vi "MemberExcuseNote.vi"() -> ()   [LabVIEW 2015, in "Member_Actor.lvlib"]
uses:
  Member_Actor.lvlib
  ExcuseNote/ExcuseNote.lvclass
  <vilib>/Utility/error.llb/Error Cluster From Error Code.vi
  <vilib>/ErrorRing/Error Ring.xnode
panel:
  in  "ExcuseNote":T1
  in  "提交":bool
  in  "Stop":bool
  out "Member_Actor.lvlib:ExcuseNote.lvclass":refnum<class "ExcuseNote.lvclass">
  in  "Member_Actor.lvlib:ExcuseNote.lvclass":refnum<class "ExcuseNote.lvclass">
  # "-"
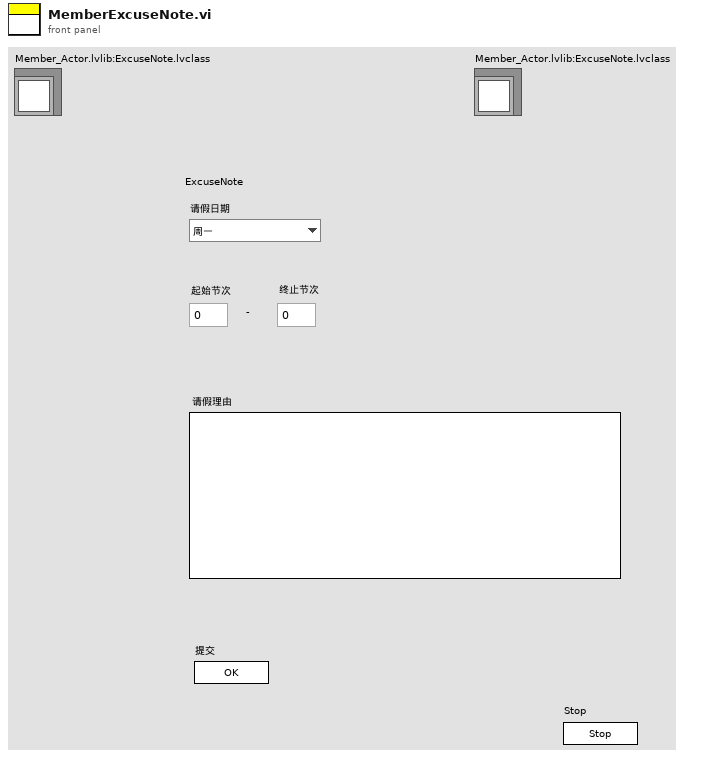
[diagram p1: front panel]
types:
  T1 = cluster{"请假日期":enum16{"周一", "周二", "周三", "周四", "周五", "周六", "周日"}, "起始节次":i32, "终止节次":i32, "请假理由":string}
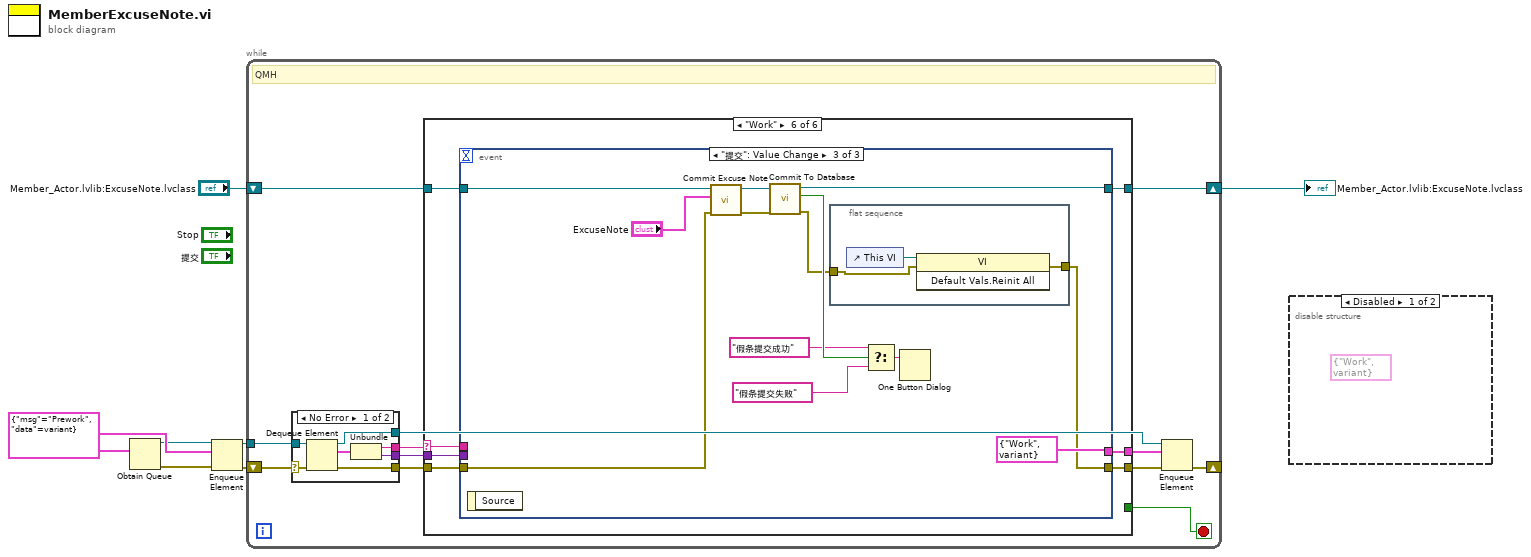
[diagram p0: block diagram]
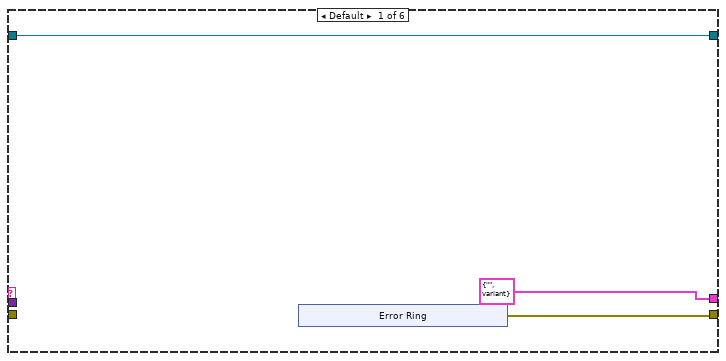
[diagram p3: hidden frame]
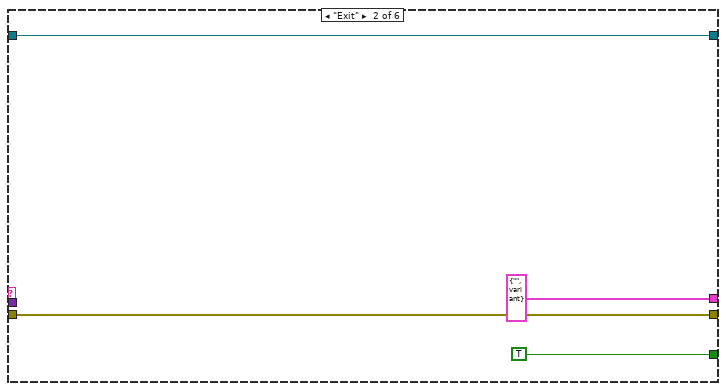
[diagram p4: hidden frame]
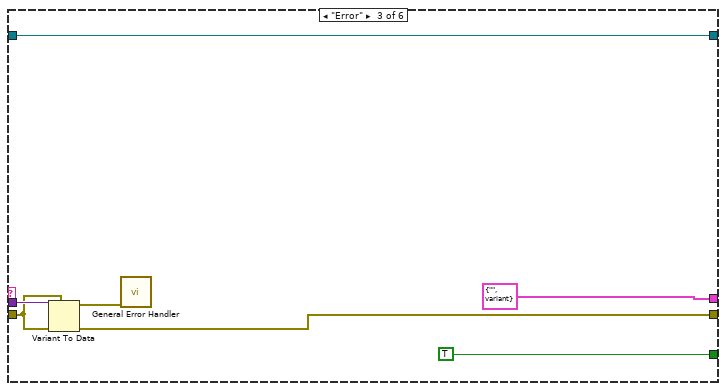
[diagram p5: hidden frame]
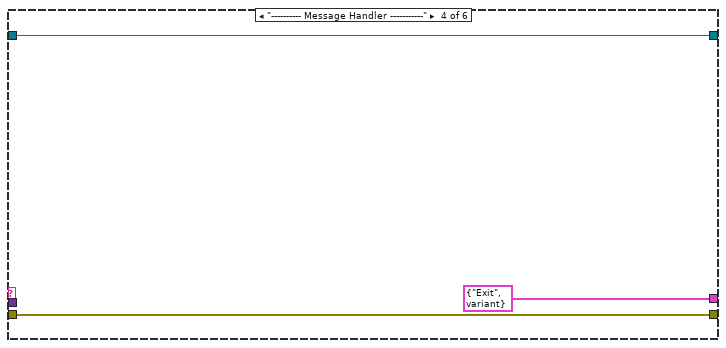
[diagram p6: hidden frame]
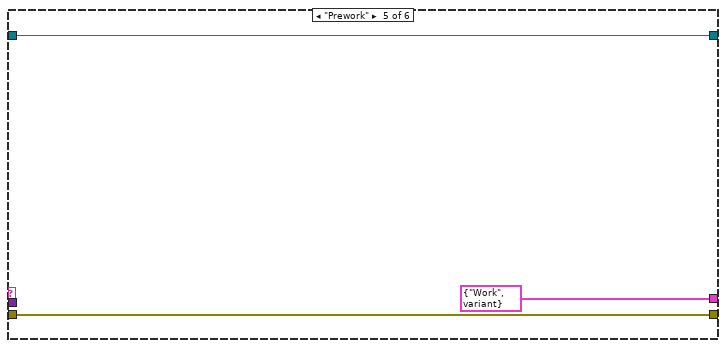
[diagram p7: hidden frame]
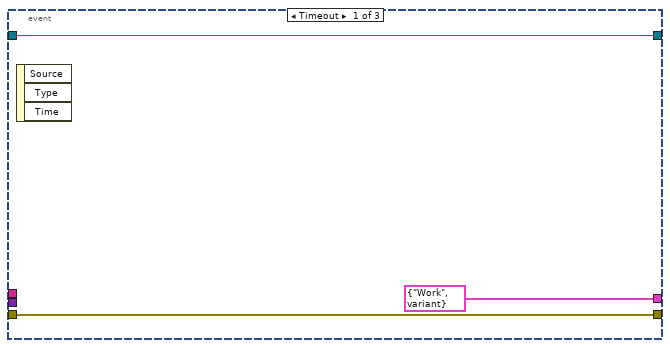
[diagram p8: hidden frame]
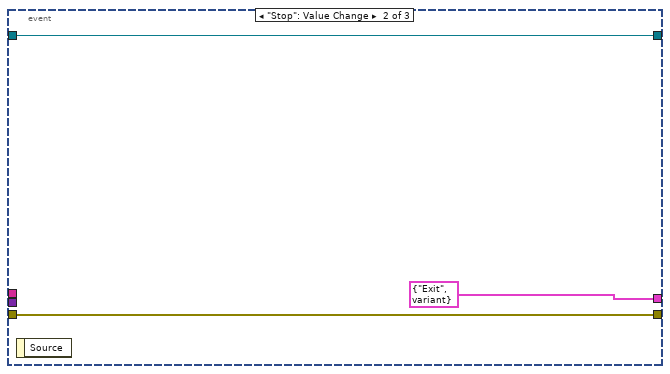
[diagram p9: hidden frame]
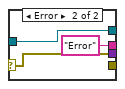
[diagram p10: hidden frame]
diagram:
  w5 = cluster{"msg":string, "data":variant} {"msg"="Prework", "data"=variant}
  n1 = Obtain Queue(element data type=w5) -> (queue out=w3:refnum<queue>, error out=w4:errorcluster)  [unwired: 4 in, 1 out]
  n2 = Enqueue Element(queue=w3, element=w5, error in (no error)=w4) -> (queue out=w6:refnum<queue>, error out=w7:errorcluster)  [unwired: 1 in, 1 out]
  n3 = while {
    tunnel: w6 -> [w18]
    shift-right: [w13] -> _
    shift-left: w7 -> [w19]
    shift-right: [w8] -> w1
    shift-left: "Member_Actor.lvlib:ExcuseNote.lvclass" -> [w9]
    stop <- w10 stop-if-true
    # "QMH"
    n4 = case shown="No Error" w19 {
      selector: w19 -> [w79 w83]
      tunnel: w18 -> [w80 w81]
      tunnel: [w78 _] -> w17
      tunnel: [w76 "Error" ("msg")] -> w16
      tunnel: [w75 w83] -> w15
      tunnel: [w74 w81] -> w12
      frame No Error {
        n5 = Dequeue Element(queue=w80, error in (no error)=w79) -> (queue out=w74:refnum<queue>, element=w77:cluster{"msg":string, "data":variant}, error out=w78:errorcluster)  [unwired: 1 in, 1 out]
        n6 = Unbundle(w77) -> ("msg"=w76:string, "data"=w75:variant)
      }
      frame Error {
      }
    }
    n7 = case shown="\"Work\"" w16 {
      selector: w16 -> [_ _ _ _ _ w49]
      tunnel: w17 -> [_ w31 w37 w41 w43 w51]
      tunnel: w15 -> [_ _ w38 _ _ w50]
      tunnel: [w22 w31 w35 w41 w43 w48] -> w14
      tunnel: [cluster{"msg":string, "data":variant} {"msg"="", "data"=variant} cluster{"msg":string, "data":variant} {"msg"="", "data"=variant} cluster{"msg":string, "data":variant} {"msg"="", "data"=variant} cluster{"msg":string, "data":variant} {"msg"="Exit", "data"=variant} cluster{"msg":string, "data":variant} {"msg"="Work", "data"=variant} w47] -> w11
      tunnel: [_ TRUE TRUE _ _ _] -> w10
      tunnel: w9 -> [w20 w28 w32 w39 w42 w46]
      tunnel: [w20 w28 w32 w39 w42 w45] -> w8
      frame Default {
        n8 = xnode "Error Ring"() -> ("error out"=w22:errorcluster)
      }
      frame "Exit" {
      }
      frame "Error" {
        n9 = Variant To Data(error in=w37, type=w37, Variant=w38) -> (data=w36:errorcluster, error out=w35:errorcluster)
        n10 = call <vilib>:"General Error Handler.vi"("error in (no error)"=w36) -> ()  [unwired: 10 in, 5 out]
      }
      frame "---------- Message Handler -----------" {
      }
      frame "Prework" {
      }
      frame "Work" {
        n11 = event shown="[2] \"提交\": Value Change" {
          selector: _ -> [_ _ _]
          dyn-events: _ -> [_ _ _]
          timeout: _ -> [_ _ _]
          tunnel: w51 -> [w54 w57 w68]
          tunnel: w50 -> [_ _ _]
          tunnel: w49 -> [_ _ _]
          tunnel: [w54 w57 w58] -> w48
          tunnel: [cluster{"msg":string, "data":variant} {"msg"="Work", "data"=variant} cluster{"msg":string, "data":variant} {"msg"="Exit", "data"=variant} cluster{"msg":string, "data":variant} {"msg"="Work", "data"=variant}] -> w47
          tunnel: w46 -> [w52 w55 w70]
          tunnel: [w52 w55 w64] -> w45
          event Timeout {
            n12 = event-data() -> ()  [unwired: 1 in, 3 out]
          }
          event "Stop": Value Change {
            n13 = event-data() -> ()  [unwired: 1 in, 1 out]
          }
          event "提交": Value Change {
            n14 = event-data() -> ()  [unwired: 1 in, 1 out]
            n15 = call "Commit Excuse Note.vi"("error in (no error)"=w68, "ExcuseNote"="ExcuseNote", "ExcuseNote in"=w70) -> ("error out"=w65:errorcluster, "ExcuseNote out"=w66:refnum<class "ExcuseNote.lvclass">)  [unwired: 7 in]
            n16 = call "Commit To Database.vi"("error in (no error)"=w65, "ExcuseNote in"=w66) -> ("error out"=w59:errorcluster, "CommitResult(True)"=w63:bool, "ExcuseNote out"=w64:refnum<class "ExcuseNote.lvclass">)  [unwired: 7 in]
            n17 = flat-sequence {
              tunnel: w59 -> [w72]
              tunnel: [w71] -> w58
              frame #0 {
                n18 = control-ref of="This VI"() -> (w73:refnum<vi>)
                n19 = invoke class="VI" method="Default Vals.Reinit All"(reference=w73, error in=w72) -> (error out=w71:errorcluster)  [unwired: 1 in, 2 out]
              }
            }
            n20 = Select(t="假条提交成功", s=w63, f="假条提交失败") -> (s? t:f=w60:string)
            n21 = One Button Dialog(message=w60) -> ()  [unwired: 1 in, 1 out]
          }
        }
      }
    }
    n22 = Enqueue Element(queue=w12, element=w11, error in (no error)=w14) -> (error out=w13:errorcluster)  [unwired: 1 in, 2 out]
  }
  "Member_Actor.lvlib:ExcuseNote.lvclass" <- w1
  n23 = disable-structure shown="Disabled" {
    frame Disabled {
      (unwired) cluster{"msg":string, "data":variant} {"msg"="Work", "data"=variant}
    }
    frame Enabled {
    }
  }
